vi "grabAcquire_action.vi"(0 "HGF_ImaqUsb":refnum<class "HGF_ImaqUsb.lvclass">, 2 "Image In":T1, 3 "Wait for Next Buffer? (Yes)":bool=TRUE, 5 "error in (no error)":errorcluster) -> (14 "dup HGF_ImaqUsb":refnum<class "HGF_ImaqUsb.lvclass">, 16 "Image Out":T1, 17 "Acquired Buffer Number":u32, 19 "error out":errorcluster)   [LabVIEW 2009, in "HGF_ImaqUsb.lvclass"]
doc: "Acquires an image from a grab acquisition. Use the grab function for high-speed image acquisition.\n\nWait parameter is ignored by IMAQ for USB."
uses:
  HGF_ImaqUsb.lvclass
  <vilib>/vision/Image Controls.llb/IMAQ Image.ctl
  HGF_ImaqUsb.lvclass/HGF_ImaqUsb.ctl
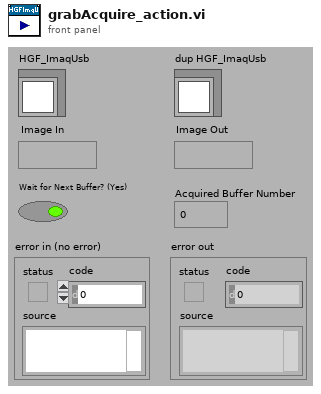
[diagram p1: front panel]
types:
  T1 = typedef "IMAQ Image.ctl" = refnum<image>
  T2 = typedef "IMAQ USB.ctl" = refnum<k1>
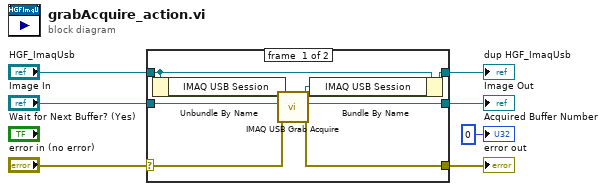
[diagram p0: block diagram]
diagram:
  n1 = case shown="No Error" "error in (no error)" {
    selector: "error in (no error)" -> [w8 w16]
    tunnel: "Image In" -> [w15 w17]
    tunnel: [w14 w17] -> w6
    tunnel: "HGF_ImaqUsb" -> [w12 w18]
    tunnel: [w10 w18] -> w4
    tunnel: [w9 w16] -> w3
    frame #0 {
      n2 = Unbundle By Name(w12) -> ("IMAQ USB Session"=w13:T2)
      n3 = call <vilib>:"IMAQ USB Grab Acquire.vi"("error in (no error)"=w8, "Image in"=w15, "IMAQ USB Session In"=w13) -> ("error out"=w9:errorcluster, "Image out"=w14:T1, "IMAQ USB Session Out"=w11:T2)  [unwired: 6 out]
      n4 = Bundle By Name(cluster=w12, "IMAQ USB Session"=w11) -> (w10:refnum<class "HGF_ImaqUsb.lvclass">)
    }
    frame #1 {
    }
  }
  "error out" <- w3
  "dup HGF_ImaqUsb" <- w4
  "Image Out" <- w6
  "Acquired Buffer Number" <- u32 0 ("Acquired Buffer Number")
